vi "日志信息主动发送(子VI).vi"   [LabVIEW 2016]
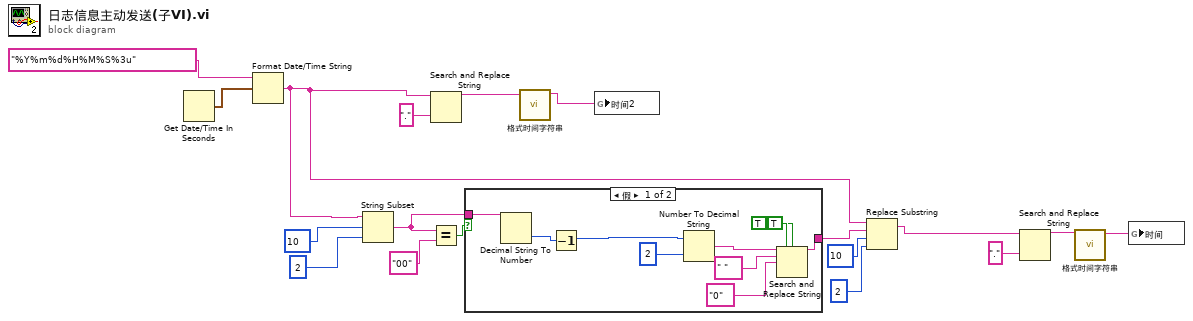
[diagram p0: block diagram]
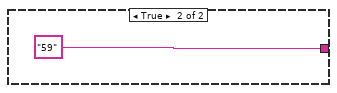
[diagram p2: hidden frame]
diagram:
  n1 = Get Date/Time In Seconds() -> (seconds since 1Jan1904=w6:timestamp)
  n2 = Format Date/Time String(time format string (%c)="%Y%m%d%H%M%S%3u" ("时间格式字符串(%c)"), seconds (now)=w6) -> (date/time string=w1:string)  [unwired: 1 in]
  n3 = String Subset(string=w1, offset (0)=10 ("偏移量(0)"), length (rest)=2 ("长度（子字符串长度）")) -> (substring=w13:string)
  n4 = Search and Replace String(input string=w1, search string="." ("搜索字符串")) -> (result string=w8:string)  [unwired: 6 in, 3 out]
  n5 = Equal?(x=w13, y="00") -> (x = y?=w12:bool)
  n6 = case shown="假" w12 {
    tunnel: w13 -> [w28 _]
    tunnel: [w20 "59" ("y")] -> w14
    frame False {
      n7 = Decimal String To Number(string=w28) -> (number=w27:i32)  [unwired: 2 in, 1 out]
      n8 = Decrement(x=w27) -> (x-1=w21:i32)
      n9 = Number To Decimal String(number=w21, width (-)=i16 2 ("宽度(-)")) -> (decimal integer string=w23:string)
      n10 = Search and Replace String(replace all?=TRUE ("替换全部？(F)"), case sensitive?=TRUE ("忽略大小写？(F)"), input string=w23, search string=" " ("搜索字符串"), replace string="0" ("替换字符串(\"\")")) -> (result string=w20:string)  [unwired: 3 in, 3 out]
    }
    frame True {
    }
  }
  n11 = call "格式时间字符串.vi"("字符串"=w8) -> ("连接的字符串"=w4:string)  [unwired: 10 in]
  n12 = global write "全局 时间2.vi" "时间2"(w4) -> ()
  n13 = Replace Substring(2:2 ("长度（子字符串长度）"), 3:10 ("偏移量(0)"), 4:w14, 5:w1) -> (1:w2:string)  [unwired: 1 out]
  n14 = Search and Replace String(input string=w2, search string="." ("搜索字符串")) -> (result string=w17:string)  [unwired: 6 in, 3 out]
  n15 = call "格式时间字符串.vi"("字符串"=w17) -> ("连接的字符串"=w3:string)  [unwired: 10 in]
  n16 = global write "全局 时间.vi" "时间"(w3) -> ()
